vi "Test_Voltage_Calc.vi"() -> ()   [LabVIEW 2025, in "phlair-busch-dilico-can-bus.lvlib"]
uses:
  phlair-busch-dilico-can-bus.lvlib
panel:
  out "Average":dbl format="%#_6f"
  out "Min":dbl
  out "Max":dbl
  out "Stack V":dbl
  in  "Number of Colum":u32
  out "Cell Array":T1(array[cluster]) {"Cell i" scale=0.0..3.0 scale format="%#_3f"}
  out "CVM":cluster{i32[], dbl[unit][]}(graph)
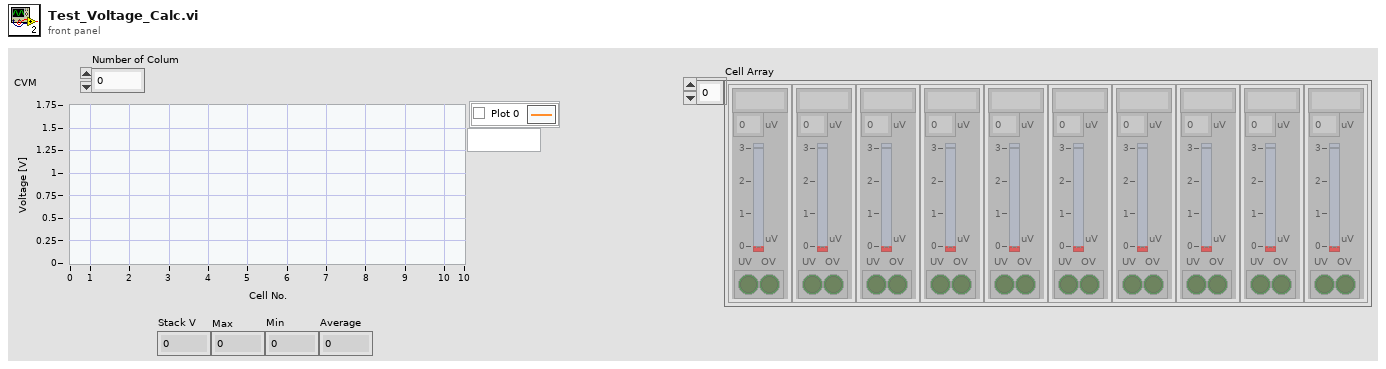
[diagram p1: front panel]
types:
  T1 = cluster{"Cell i":string, "Cell i":dbl[unit], " UV   OV ":bool[]}[]
  T2 = cluster{"Cell i":string, "Cell U":dbl[unit], " UV   OV ":bool[]}[]
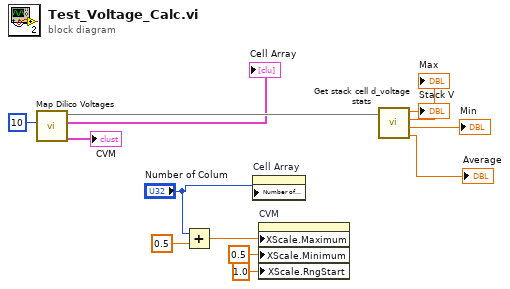
[diagram p0: block diagram]
diagram:
  n1 = call "Map Dilico Voltages.vi"("#Cell Request"=u8 10) -> ("CVM"=→"CVM":cluster{i32[], dbl[unit][]}, "Cell Array"=→"Cell Array":T2, "Dilico Values"=w13:map{string, dbl})  [unwired: 7 in, 1 out]
  n2 = Add(x="Number of Colum", y=0.5) -> (x+y=w9:dbl)
  n3 = property on="Cell Array" class="Arr (strict)"("Number of Columns"="Number of Colum") -> ()  [unwired: 2 in, 2 out]
  n4 = property on="CVM" class="XYGraph (strict)"("XScale.Maximum"=w9, "XScale.Minimum"=0.5 ("X Scale.Range:Minimum"), "XScale.RngStart"=1.0 ("X Scale.Range:Start")) -> ()  [unwired: 2 in, 2 out]
  n5 = call "Get stack cell d_voltage stats.vi"("Status Map"=w13) -> ("Average"=→"Average":dbl, "Min"=→"Min":dbl, "Max"=→"Max":dbl, "Stack V"=→"Stack V":dbl)  [unwired: 7 in]
